vi "BRig_dataMTrig_SolenoidCal_N.vi"() -> (2 "output_SolenoidCal_N":i32)   [LabVIEW 2014]
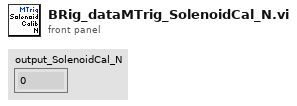
[diagram p1: front panel]
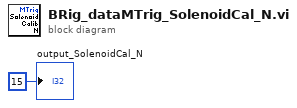
[diagram p0: block diagram]
diagram:
  "output_SolenoidCal_N" <- 15 ("output_iBlock")
